vi "PostgreSQL EC2 Example.vi"() -> ()   [LabVIEW 2020]
uses:
  Data.PG/Data.PG.lvclass
panel:
  out "Result":string[][](array[string])
  in  "command":string="SELECT * FROM test_table where my_dbl>0.99;"
  in  "error in (no error)":errorcluster
  in  "connection info":T1={"host"="ec2-3-15-178-117.us-east-2.compute.amazonaws.com", "port"="5432", "user"="postgres", "dbname"="postgres", "password"=""}
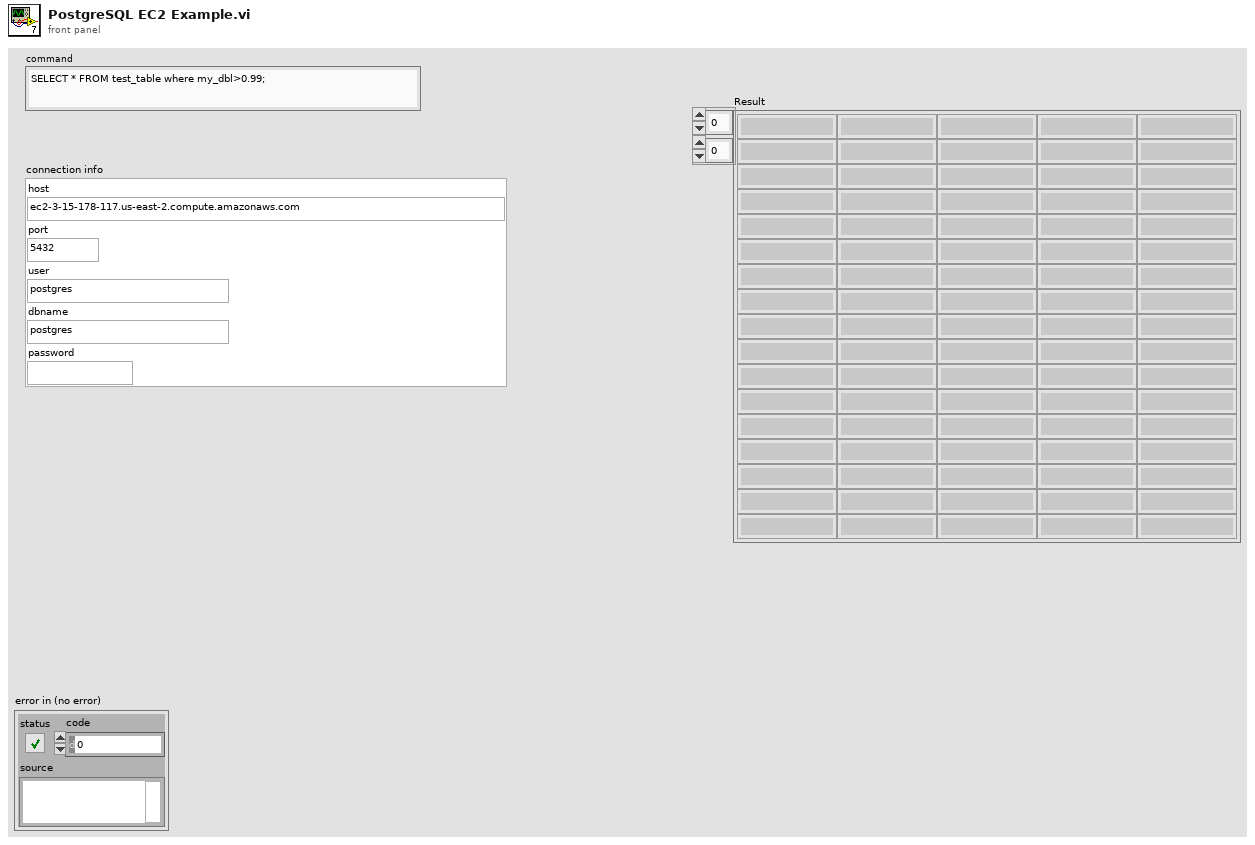
[diagram p1: front panel]
types:
  T1 = cluster{"host":string, "port":string, "user":string, "dbname":string, "password":string}
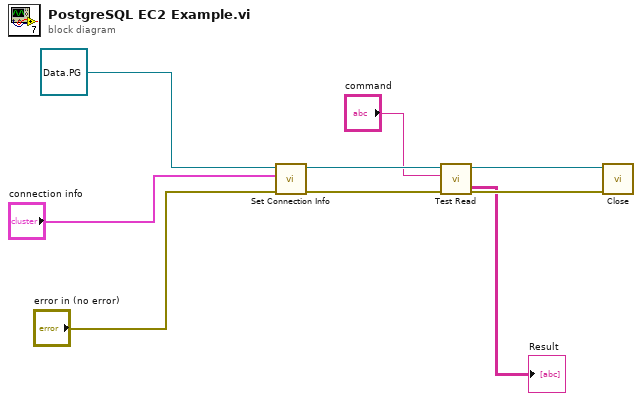
[diagram p0: block diagram]
diagram:
  n1 = call "Set Connection Info.vi"("error in (no error)"="error in (no error)", "connection info"="connection info", "Data.PG in"=refnum<class "Data.PG.lvclass"> refnum) -> ("error out"=w5:errorcluster, "Data.PG out"=w6:refnum<class "Data.PG.lvclass">)  [unwired: 7 in]
  n2 = call-dynamic "Test Read.vi"("error in (no error)"=w5, "command"="command", "Data.PG in"=w6) -> ("error out"=w3:errorcluster, "Data.PG out"=w4:refnum<class "Data.PG.lvclass">, "Result"=→"Result":string[][])  [unwired: 3 in, 3 out]
  n3 = call-dynamic "Close.vi"("error in (no error)"=w3, "Data.PG in"=w4) -> ()  [unwired: 8 in, 2 out]
